vi "SUB_ReadScript_File.vi"(0 "Script FileName":string) -> (2 "text":string, 3 "error out":errorcluster, 4 "path string":string)   [LabVIEW 2011]
panel:
  out "path":path
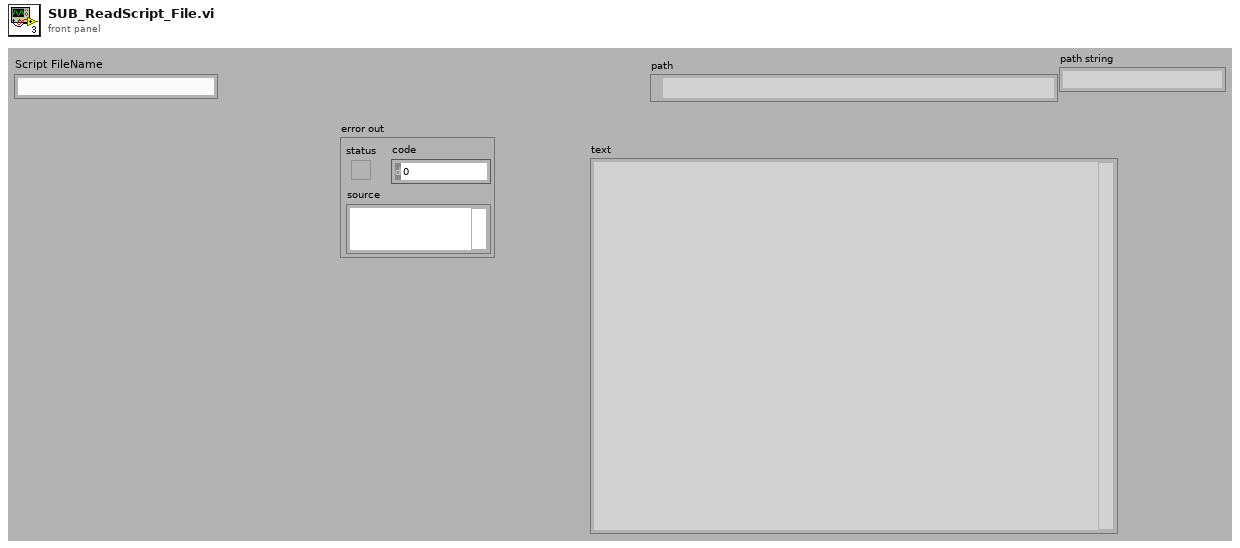
[diagram p1: front panel]
types:
  T1 = enum32{"invalid app kind", "Development System", "Run Time System", "Student Edition", "Embedded LabVIEW", "Evaluation", "Custom"}
  T2 = enum16{"open", "replace", "create", "open or create", "replace or create", "replace or create with confirmation"}
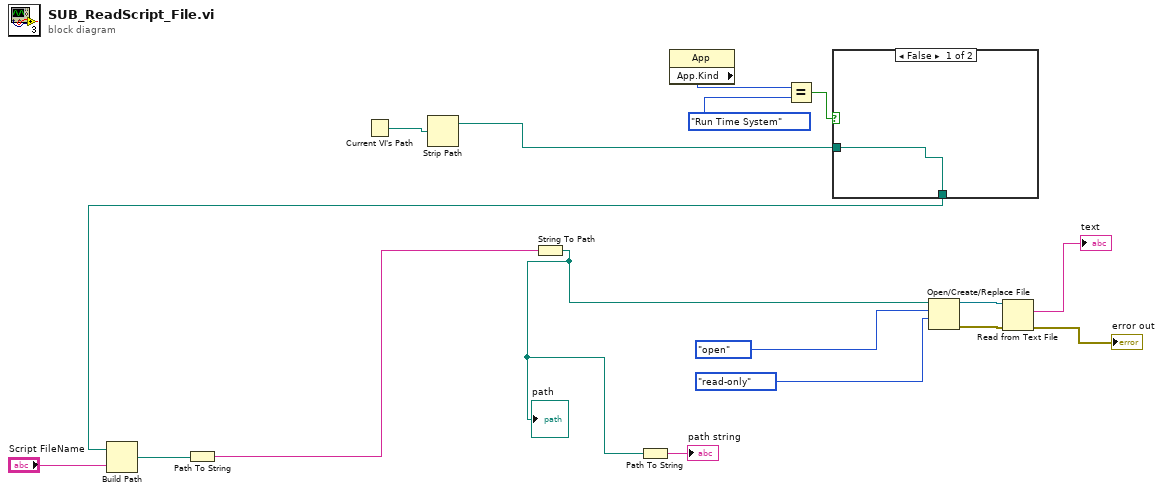
[diagram p0: block diagram]
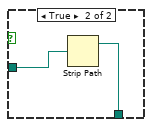
[diagram p2: hidden frame]
diagram:
  n1 = Current VI's Path() -> (path=w11:path)
  n2 = Strip Path(path=w11) -> (stripped path=w7:path)  [unwired: 1 out]
  n3 = property class="App"() -> ("App.Kind"=w10:T1)  [unwired: 2 in, 2 out]
  n4 = Equal?(x=w10, y=T1."Run Time System" ("Application:Kind")) -> (x = y?=w8:bool)
  n5 = case shown="False" w8 {
    tunnel: w7 -> [w18 w20]
    tunnel: [w18 w19] -> w5
    frame False {
    }
    frame True {
      n6 = Strip Path(path=w20) -> (stripped path=w19:path)  [unwired: 1 out]
    }
  }
  n7 = Build Path(base path=w5, name or relative path="Script FileName") -> (appended path=w6:path)
  n8 = Path To String(path=w6) -> (string=w4:string)
  n9 = String To Path(string=w4) -> (path=w2:path)
  "path" <- w2
  n10 = Path To String(path=w2) -> (string=→"path string":string)
  n11 = Open/Create/Replace File(file path (use dialog)=w2, operation (0:open)=T2."open", access (0:read/write)=enum16{"read/write", "read-only", "write-only"}."read-only") -> (refnum out=w15:refnum<file>, error out=w14:errorcluster)  [unwired: 3 in, 1 out]
  n12 = Read from Text File(file (use dialog)=w15, error in=w14) -> (text=→"text":string, error out=→"error out":errorcluster)  [unwired: 2 in, 2 out]
